vi "GetRealAndImageSubVI).vi"(10 "byte data":u8 format="%x", 11 "sn":string) -> (3 "output frame":string)   [LabVIEW 2012]
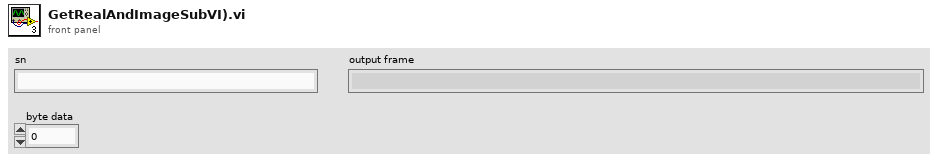
[diagram p1: front panel]
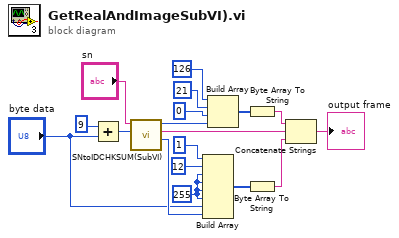
[diagram p0: block diagram]
diagram:
  w12 = u8 255
  n1 = Add(x=u8 9, y="byte data") -> (x+y=w14:u8)
  n2 = call "SNtoIDCHKSUM(SubVI).vi"("fix cheksum"=w14, "input sn"="sn") -> ("output check sum"=w16:u8, "output sn"=w9:string, "output id"=w8:u8)  [unwired: 7 in]
  n3 = Build Array(u8 1, u8 12, w12, w12, w12, w12, "byte data", w16) -> (w17:u8[])
  n4 = Build Array(u8 126, u8 21, u8 0, w8) -> (w2:u8[])
  n5 = Byte Array To String(unsigned byte array=w2) -> (string=w3:string)
  n6 = Byte Array To String(unsigned byte array=w17) -> (string=w18:string)
  n7 = Concatenate Strings(w3, w9, w18) -> (→"output frame":string)
